vi "GetEUIEvents.vi"(8 "error in (no error)":errorcluster, 11 "Model in":refnum<class "Model.lvclass">) -> (0 "error out":errorcluster, 2 "EUI Events out":refnum<class "EUI Events.lvclass">, 3 "Model out":refnum<class "Model.lvclass">)   [LabVIEW 2016, in "Model.lvclass"]
uses:
  Model.lvclass
  EUI Events/EUI Events.lvclass
  Model.lvclass/Model.ctl
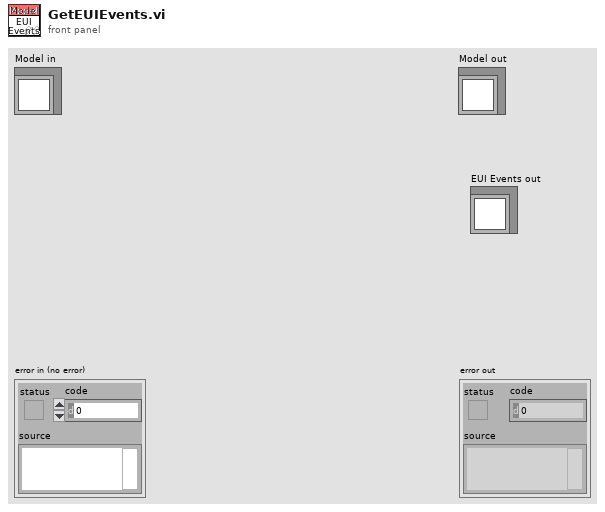
[diagram p1: front panel]
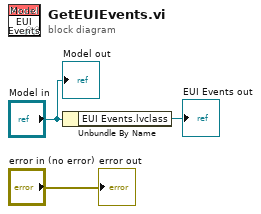
[diagram p0: block diagram]
diagram:
  n1 = Unbundle By Name("Model in") -> ("EUI Events.lvclass"=→"EUI Events out":refnum<class "EUI Events.lvclass">)
  "error out" <- "error in (no error)"
  "Model out" <- "Model in"
